vi "Index Testing.vi"() -> ()   [LabVIEW 2021]
uses:
  <vilib>/Modbus/master/Create Master Instance (Serial).vi
  <vilib>/Modbus/master/Modbus Master.lvclass
panel:
  out "register values":u16[](array[numeric])
  in  "Index":bool[](array[boolean])
  out "error out 6":errorcluster
  out "error out 5":errorcluster
  out "error out 4":errorcluster
  out "error out 3":errorcluster
  out "error out 2":errorcluster
  out "error out":errorcluster
  in  "stop":bool
  in  "Tarhet Position":i32=28800683
  in  "Index S.T.L":u16=300
  in  "Index H.T.L":u16=300
  out "Index Status":bool[](array[boolean])
  # "Index\nStart Index\nReset Index"
  # "Running"
  # "Completed"
  # "Error"
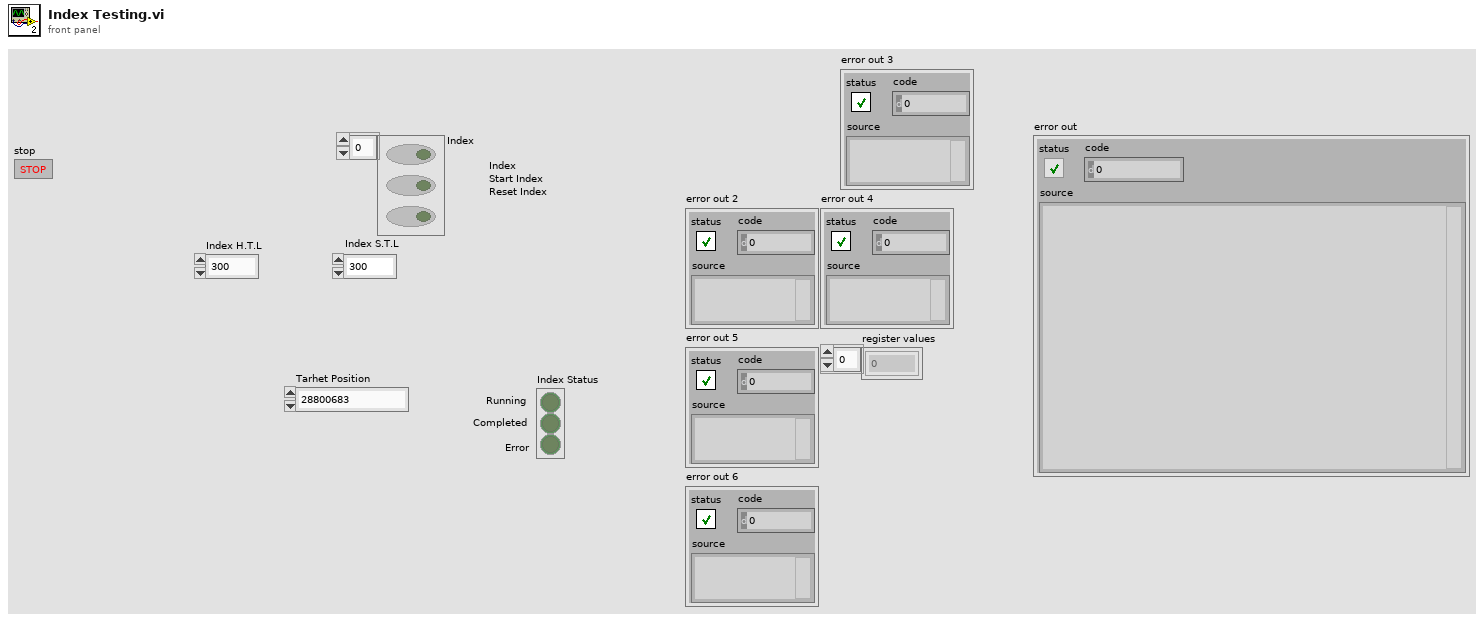
[diagram p1: front panel]
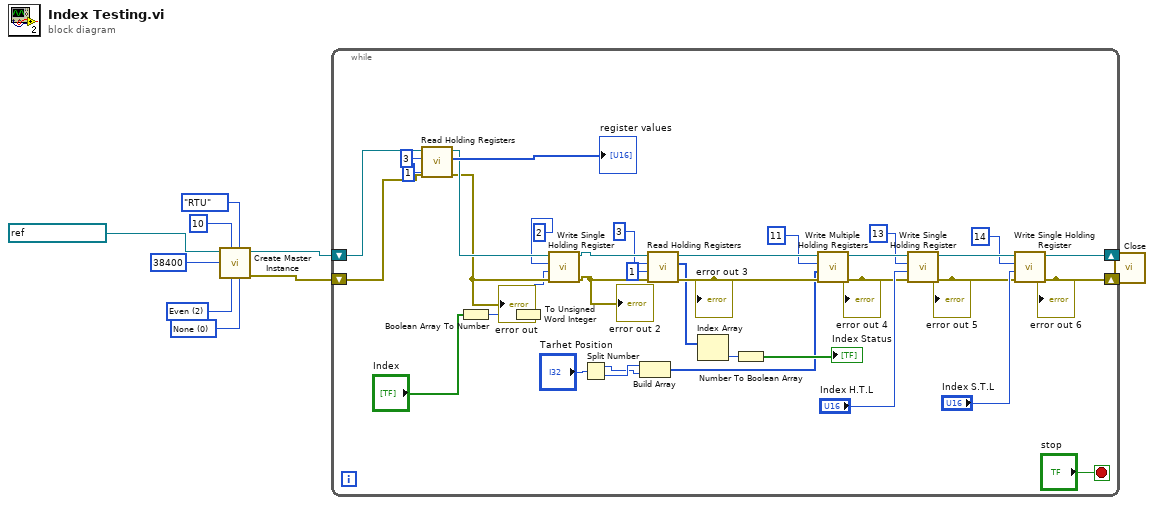
[diagram p0: block diagram]
diagram:
  w8 = u16 0 items=["None", "XON/XOFF", "RTS/CTS", "XON/XOFF & RTS/CTS", "DTR/DSR", "XON/XOFF & DTR/DSR"] ("flow control (None)")
  w9 = u16 2 items=["None", "Odd", "Even"] ("parity (Even)")
  n1 = call-poly <vilib>:"Create Master Instance.vi"("flow control (None)"=w8, "serial type"=enum16{"RTU", "ASCII"}."RTU", "parity (Even)"=w9, "unit ID"=u8 10, "baud rate (9600)"=u32 38400, "VISA resource name"=refnum<visa-resource-name> "ASRL1::INSTR") -> ("error out"=w5:errorcluster, "serial master instance"=w4:refnum<class "Modbus Master.lvclass">)  [unwired: 4 in]
  n2 = while {
    shift-right: [w45] -> w2
    shift-left: w5 -> [w38]
    shift-right: [w46] -> w3
    shift-left: w4 -> [w39]
    stop <- "stop" stop-if-true
    n3 = call-dynamic "Read Holding Registers.vi"("error in (no error)"=w38, "number of holding registers"=u16 1, "starting address"=u16 3, "Modbus master in"=w39) -> ("error out"=w33:errorcluster, "register values"=→"register values":u16[], "Modbus master out"=w34:refnum<class "Modbus Master.lvclass">)  [unwired: 5 in]
    "error out" <- w33
    n4 = Boolean Array To Number(Boolean array="Index") -> (number=w31:u32)
    n5 = To Unsigned Word Integer(number=w31) -> (unsigned 16bit integer=w30:u16)
    n6 = call-dynamic "Write Single Holding Register.vi"("error in (no error)"=w33, "holding register value"=w30, "address"=u16 2, "Modbus master in"=w34) -> ("error out"=w42:errorcluster, "Modbus master out"=w43:refnum<class "Modbus Master.lvclass">)  [unwired: 6 in]
    "error out 2" <- w42
    n7 = Split Number(x="Tarhet Position") -> (hi(x)=w11:u16, lo(x)=w12:u16)
    n8 = Build Array(w12, w11) -> (w20:u16[])
    n9 = call-dynamic "Read Holding Registers.vi"("error in (no error)"=w42, "number of holding registers"=u16 1, "starting address"=u16 3, "Modbus master in"=w43) -> ("error out"=w28:errorcluster, "register values"=w25:u16[], "Modbus master out"=w27:refnum<class "Modbus Master.lvclass">)  [unwired: 5 in]
    "error out 3" <- w28
    n10 = Index Array(array=w25) -> (element=w24:u16)  [unwired: 1 in]
    n11 = Number To Boolean Array(number=w24) -> (Boolean array=→"Index Status":bool[])
    n12 = call-dynamic "Write Multiple Holding Registers.vi"("error in (no error)"=w28, "holding register values"=w20, "starting address"=u16 11, "Modbus master in"=w27) -> ("error out"=w17:errorcluster, "Modbus master out"=w18:refnum<class "Modbus Master.lvclass">)  [unwired: 6 in]
    "error out 4" <- w17
    n13 = call-dynamic "Write Single Holding Register.vi"("error in (no error)"=w17, "holding register value"="Index H.T.L", "address"=u16 13, "Modbus master in"=w18) -> ("error out"=w15:errorcluster, "Modbus master out"=w16:refnum<class "Modbus Master.lvclass">)  [unwired: 6 in]
    "error out 5" <- w15
    n14 = call-dynamic "Write Single Holding Register.vi"("error in (no error)"=w15, "holding register value"="Index S.T.L", "address"=u16 14, "Modbus master in"=w16) -> ("error out"=w45:errorcluster, "Modbus master out"=w46:refnum<class "Modbus Master.lvclass">)  [unwired: 6 in]
    "error out 6" <- w45
  }
  n15 = call-dynamic "Close.vi"("error in (no error)"=w2, "Modbus master in"=w3) -> ()  [unwired: 9 in, 1 out]
